vi "全局1.vi"() -> ()   [LabVIEW 2016]
panel:
  in  "枚举":enum16{"返回请求应答", "上传数据", "返回执行结果"}(ring)
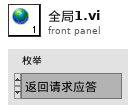
[diagram p1: front panel]
diagram:
